vi "配置属性写入.vi"(4 "error in (no error)":errorcluster caption="错误输入（无错误）", 5 "Value":u8(ring) items=["三通阀", "排阀"], 6 "Container State":T2 caption="容器状态", 7 "Display State In":T1 caption="显示状态输入" {"值" items=["三通阀", "排阀"]}) -> (0 "error out":errorcluster caption="错误输出", 3 "Display State Out":T1 caption="显示状态输出" {"值" items=["三通阀", "排阀"]})   [LabVIEW 2016, in "CODMn调试控件V3.xctl"]
uses:
  <vilib>/_xctls/Container State.ctl
  <vilib>/_xctls/XControlSupport.lvlib
panel:
  # "将以下值显示控件替换为所需类型的显示控件。\n不要从连线板中删除该显示控件或其它显示控件。\n不要更改连线板模式。\n值显示控件应始终位于连线板输出端自顶部起第三个接线端。"
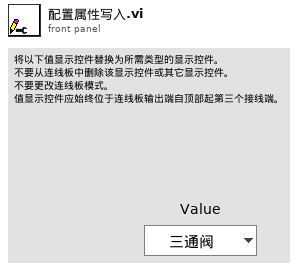
[diagram p1: front panel]
types:
  T1 = typedef "CODMn调试控件V3.xctl/状态 2.ctl" = cluster{"值":u8}
  T2 = typedef "XControlSupport.lvlib/Container State.ctl" = cluster{"Indicator?":bool, "Run Mode?":bool, " Refnum":refnum<vi>}
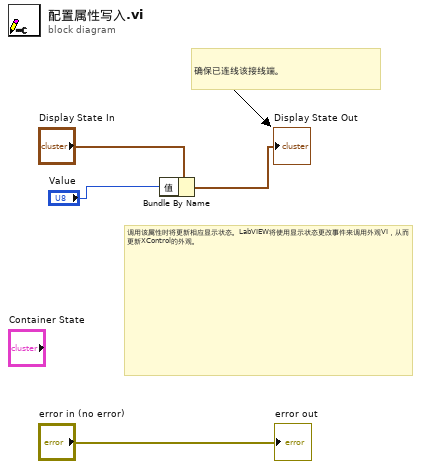
[diagram p0: block diagram]
diagram:
  # "确保已连线该接线端。"
  # "调用该属性时将更新相应显示状态。LabVIEW将使用显示状态更改事件来调用外观VI，从而更新XControl的外观。"
  n1 = Bundle By Name(cluster="Display State In", "值"="Value") -> (→"Display State Out":T1)
  "error out" <- "error in (no error)"
